vi "Example_Host SPI Dual Port.vi"() -> ()   [LabVIEW 2019]
uses:
  Host API/Controls/SPI Configuration Cluster.ctl
  <vilib>/FPGAPlugInAG/myRIO-1900/niLvFpga_Open_myRIO-1900.vi
  <vilib>/Utility/error.llb/Error Cluster From Error Code.vi
  <vilib>/RVI Host/nirviSupport.llb/nirviErrorClusterFromErrorCode.vi
  <vilib>/rvi/errors/niLvFpgaAdjustHostInterfaceError.vi
  <vilib>/FPGAPlugInAG/myRIO-1900/niLvFpga_Close_myRIO-1900.vi
  <vilib>/rvi/interface/nirviOpenFPGA/nirviOpenFPGA.xnode
  Host API/Controls/FPGA Reference.ctl
  FPGA Bitfiles/SPIExample_FPGATarget2_FPGASPIFPGATopLe_zKpK3F1T2ns.lvbitx
  <vilib>/rvi/interface/nirviMethod/nirviMethod.xnode
  <vilib>/rvi/interface/nirviCloseFPGA/nirviCloseFPGA.xnode
  <vilib>/rvi/interface/nirviMethod/StockFPGA_InlinedMethodWaitForSingleIRQ.vi
  <vilib>/FPGAPlugInAG/myRIO-1900/niLvFpga_WaitOnIrq_myRIO-1900.vi
  <vilib>/FPGAPlugInAG/myRIO-1900/niLvFpga_AcknowledgeIrq_myRIO-1900.vi
panel:
  out "Thermometer":dbl(slide) scale=0.0..100.0
  in  "Total Bits":u16=8
  in  "Configuration Cluster":T1={"CS"=1, "Clock Rate (Hz)"=50000.0, "Clock Mode"=0, "CS Active State"=FALSE} {"CS" items=["0"=1, "1"=2, "2"=4, "3"=8, "4"=16, "5"=32, "6"=64, "7"=128]; "Clock Mode" items=["0", "1", "2", "3"]}
  in  "Port":i8
  in  "Write":bool
  in  "Write Data":u8[](array[numeric])
  in  "stop":bool
  out "error out":errorcluster
  out "Read Data":u8[](array[numeric])
  # "Configure SPI"
  # "Write SPI"
  # "Control and Status"
  # "Read SPI"
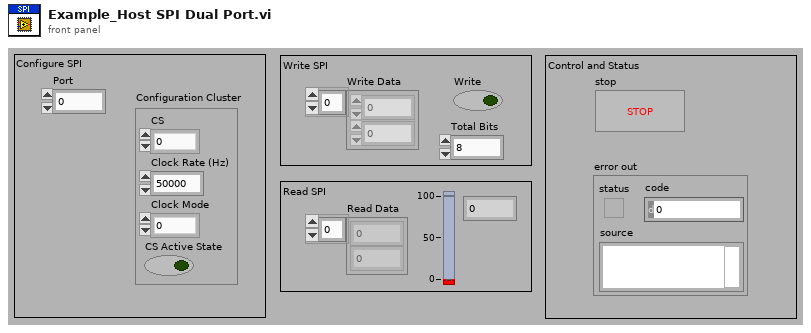
[diagram p1: front panel]
types:
  T1 = typedef "SPI Configuration Cluster.ctl" = cluster{"CS":u8, "Clock Rate (Hz)":dbl, "Clock Mode":u8, "CS Active State":bool}
  T2 = typedef "FPGA Reference.ctl" = refnum<k20>
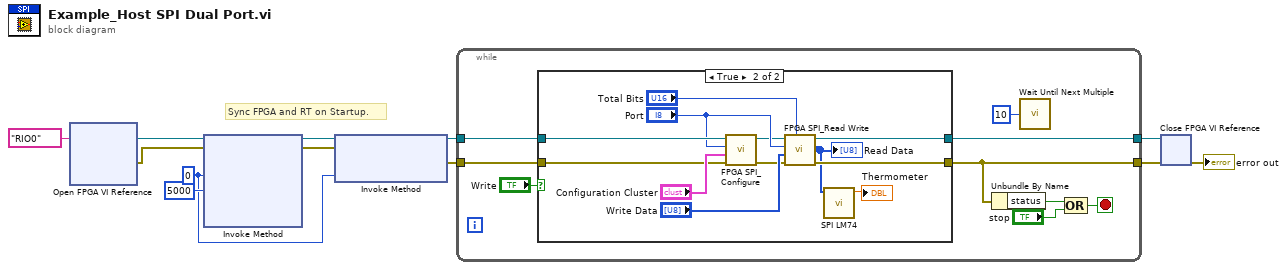
[diagram p0: block diagram]
diagram:
  w2 = 0 ("IRQ Number(s)")
  # "Sync FPGA and RT on Startup."
  n1 = xnode "Open FPGA VI Reference"("resource name"=tag "RIO0") -> ("FPGA VI Reference Out"=w9:T2, "error out"=w8:errorcluster)  [unwired: 1 in]
  n2 = xnode "Invoke Method"("FPGA VI Reference In"=w9, "error in"=w8, "IRQ Number(s)"=w2, "Timeout (ms)"=5000) -> ("FPGA VI Reference Out"=w7:T2, "error out"=w6:errorcluster)  [unwired: 2 out]
  n3 = xnode "Invoke Method"("FPGA VI Reference In"=w7, "error in"=w6, "IRQ Number(s)"=w2) -> ("FPGA VI Reference Out"=w4:T2, "error out"=w3:errorcluster)
  n4 = while {
    tunnel: w4 -> [w21]
    tunnel: w3 -> [w20]
    tunnel: [w19] -> w12
    tunnel: [w18] -> w11
    stop <- w15 stop-if-true
    n5 = case shown="True" "Write" {
      tunnel: w21 -> [w22 w30]
      tunnel: w20 -> [w23 w27]
      tunnel: [w22 w35] -> w19
      tunnel: [w23 w34] -> w18
      frame False {
      }
      frame True {
        n6 = call "FPGA SPI_Configure.vi"("error in"=w27, "Configuration Cluster"="Configuration Cluster", "Port"="Port", "FPGA VI Reference"=w30) -> ("error out"=w26:errorcluster, "FPGA VI Reference Out"=w28:T2)  [unwired: 6 out]
        n7 = call "FPGA SPI_Read Write.vi"("Total Bits"="Total Bits", "error in"=w26, "Write Data"="Write Data", "Port"="Port", "FPGA VI Reference"=w28) -> ("error out"=w34:errorcluster, "Read Data"=w25:u8[], "FPGA VI Reference Out"=w35:T2)  [unwired: 4 out]
        "Read Data" <- w25
        n8 = call "SPI LM74.vi"("array"=w25) -> ("°C"=→"Thermometer":dbl)  [unwired: 10 in]
      }
    }
    n9 = Unbundle By Name(w18) -> ("status"=w17:bool)
    n10 = call "Wait Until Next Multiple"("Count(mSec)"=u32 10) -> ()  [unwired: 1 out]
    n11 = Compound Arithmetic op=OR(w17, "stop") -> (w15:bool)
  }
  n12 = xnode "Close FPGA VI Reference"("FPGA VI Reference In"=w12, "error in"=w11) -> ("error out"=→"error out":errorcluster)
